vi "Grab Stamp Precheck.vi"(8 "error in (no error)":errorcluster, 10 "Stamp Number":i32, 11 "GrabberTool Class in":refnum<class "GrabberTool Class.lvclass">) -> (0 "error out":errorcluster, 3 "GrabberTool Class out":refnum<class "GrabberTool Class.lvclass">)   [LabVIEW 2011, in "GrabberTool Class.lvclass"]
uses:
  GrabberTool Class.lvclass
  GrabberTool Class.lvclass/GrabberTool Class.ctl
  WorkTable Class/WorkTable Class.lvclass
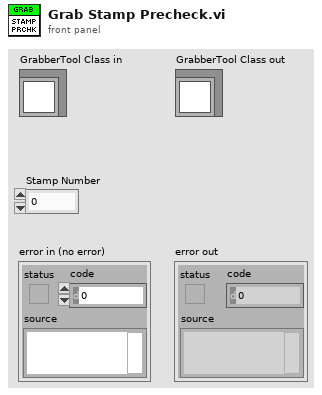
[diagram p1: front panel]
types:
  T1 = typedef "Worktable_Stamps.ctl" = cluster{"Stamp Slots":T2[], "Vacuum Channel":i32}
  T2 = typedef "Worktable_Stamp.ctl" = cluster{"Stamp State":enum16{"Empty", "Populated", "Used"}, "Location/Orientation":T3, "Stamp Type":T4}
  T3 = typedef "Position_Orientation.ctl" = cluster{"Center":refnum<class "Vec3d Class.lvclass">, "Orientation":refnum<class "Orient3d Class.lvclass">}
  T4 = typedef "Stamp Type.ctl" = enum16{"Stamp 1", "Stamp 2", "Stamp 3", "Stamp 4"}
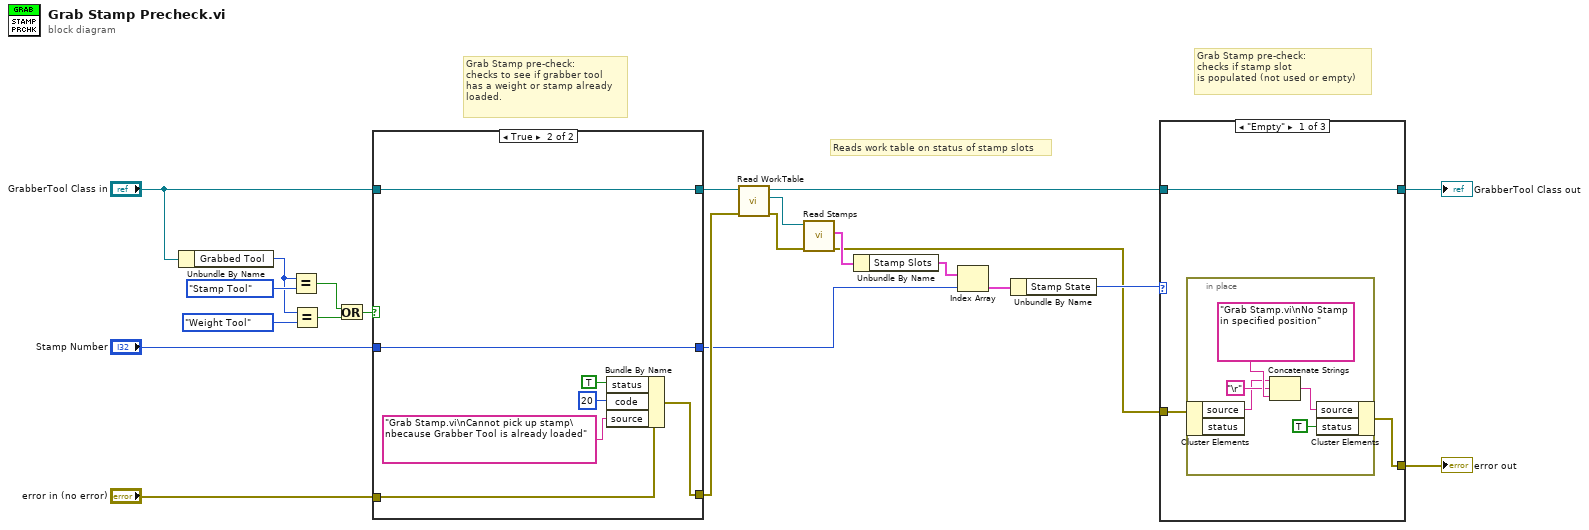
[diagram p0: block diagram]
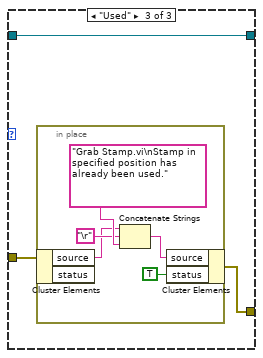
[diagram p3: hidden frame]
diagram:
  # "Reads work table on status of stamp slots"
  # "Grab Stamp pre-check:\nchecks if stamp slot\nis populated (not used or empty)"
  # "Grab Stamp pre-check:\nchecks to see if grabber tool\nhas a weight or stamp already \nloaded."
  n1 = Unbundle By Name("GrabberTool Class in") -> ("Grabbed Tool"=w16:enum16{"Weight Tool", "Stamp Tool", "Nothing"})
  n2 = Equal?(x=w16, y=enum16{"Weight Tool", "Stamp Tool", "Nothing"}."Stamp Tool") -> (x = y?=w18:bool)
  n3 = Equal?(x=w16, y=enum16{"Weight Tool", "Stamp Tool", "Nothing"}."Weight Tool") -> (x = y?=w17:bool)
  n4 = Or(x=w18, y=w17) -> (x .or. y?=w19:bool)
  n5 = case shown="True" w19 {
    tunnel: [w25 w32] -> w14
    tunnel: "GrabberTool Class in" -> [w25 w32]
    tunnel: [w24 w30] -> w13
    tunnel: "error in (no error)" -> [w24 w31]
    tunnel: [w23 w26] -> w7
    tunnel: "Stamp Number" -> [w23 w26]
    frame False {
    }
    frame True {
      n6 = Bundle By Name(cluster=w31, "status"=TRUE, "code"=20, "source"="Grab Stamp.vi\nCannot pick up stamp\nbecause Grabber Tool is already loaded") -> (w30:errorcluster)
    }
  }
  n7 = call-dynamic "Read WorkTable.vi"("error in"=w13, "Gantry Class in"=w14) -> ("error out"=w11:errorcluster, "WorkTable Class.lvclass"=w12:refnum<class "WorkTable Class.lvclass">, "Gantry Class out"=w4:refnum<class "GrabberTool Class.lvclass">)  [unwired: 7 in]
  n8 = call-dynamic "Read Stamps.vi"("error in (no error)"=w11, "WorkTable Class in"=w12) -> ("error out"=w2:errorcluster, "Stamps"=w10:T1)  [unwired: 7 in, 1 out]
  n9 = Unbundle By Name(w10) -> ("Stamp Slots"=w9:T2[])
  n10 = Index Array(array=w9, index=w7) -> (element=w6:T2)
  n11 = Unbundle By Name(w6) -> ("Stamp State"=w5:enum16{"Empty", "Populated", "Used"})
  n12 = case shown="\"Empty\"" w5 {
    tunnel: w4 -> [w35 w42 w43]
    tunnel: [w35 w42 w43] -> w3
    tunnel: w2 -> [w34 w41 w45]
    tunnel: [w33 w41 w44] -> w1
    frame "Empty" {
      n13 = in-place {
        n14 = in-place-cluster #1(w34) -> ("source"=w37:string)  [unwired: 1 out]
        n15 = Concatenate Strings(w37, "\r", "Grab Stamp.vi\nNo Stamp in specified position" ("string")) -> (w38:string)
        n16 = in-place-cluster #1("source"=w38, "status"=TRUE) -> (w33:errorcluster)
      }
    }
    frame "Populated" {
    }
    frame "Used" {
      n17 = in-place {
        n18 = in-place-cluster #2(w45) -> ("source"=w47:string)  [unwired: 1 out]
        n19 = Concatenate Strings(w47, "\r", "Grab Stamp.vi\nStamp in specified position has already been used." ("string")) -> (w48:string)
        n20 = in-place-cluster #2("source"=w48, "status"=TRUE) -> (w44:errorcluster)
      }
    }
  }
  "error out" <- w1
  "GrabberTool Class out" <- w3
